vi "JSON to LVObject.vi"(7 "Class 1 in":refnum<class "Serializer-Palette.lvclass">, 8 "error in":errorcluster, 9 "Object Type":refnum<class>, 10 "Offset":i32, 11 "JSON":string) -> (0 "error out":errorcluster, 1 "Object":refnum<class>)   [LabVIEW 2021, in "TSC Material Theme.lvlib" / "Serializer-Palette.lvclass"]
doc: "Convert JSON to an Object of a LabVIEW Class."
uses:
  Serializer-Palette.lvclass
  Serializer-Palette.lvclass/Serializer-Palette.ctl
  TSC Material Theme/material json palette--cluster.ctl
  Material-Palette/Material-Palette.lvclass/Material-Palette.ctl
  TSC Material Theme/convert string to hex.vi
  Material-Palette/Material-Palette.lvclass
  <vilib>/JDP Science/JSONtext/JSONtext.lvlib
  TSC Material Theme/TSC Material Theme.lvlib
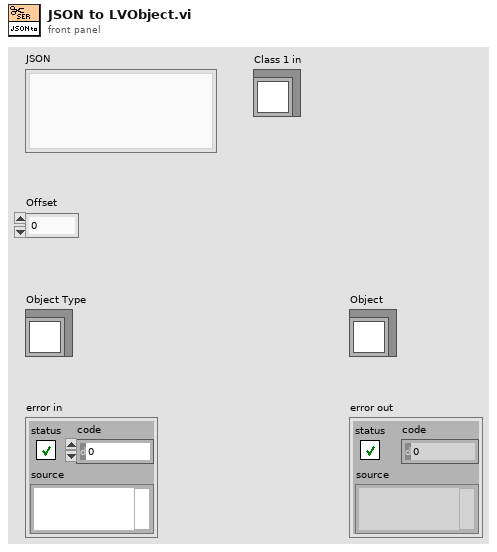
[diagram p1: front panel]
types:
  T1 = typedef "TSC Material Theme.lvlib/material json palette--cluster.ctl" = cluster{"0":string, "5":string, "10":string, "15":string, "20":string, "25":string, "30":string, "35":string, "40":string, "50":string, "60":string, "70":string, "80":string, "90":string, "95":string, "98":string, "99":string, "100":string}
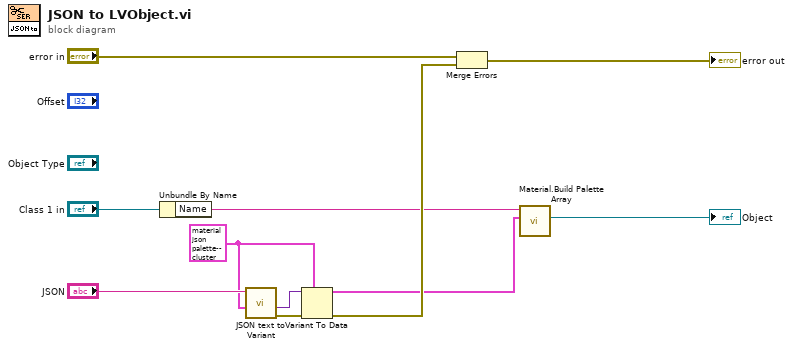
[diagram p0: block diagram]
diagram:
  w5 = T1 {"0"="", "5"="", "10"="", "15"="", "20"="", "25"="", "30"="", "35"="", "40"="", "50"="", "60"="", "70"="", "80"="", "90"="", "95"="", "98"="", "99"="", "100"=""} ("primary")
  n1 = Unbundle By Name("Class 1 in") -> ("Name"=w1:string)
  n2 = call <vilib>:"JSON text to Variant.vi"("Data Type"=w5, "JSON"="JSON") -> ("error out"=w11:errorcluster, "Variant out"=w6:variant)  [unwired: 8 in]
  n3 = Variant To Data(error in=w11, type=w5, Variant=w6) -> (data=w2:T1, error out=w9:errorcluster)
  n4 = Merge Errors("error in", w9) -> (→"error out":errorcluster)
  n5 = call "Material.Build Palette Array.vi"("palette"=w2, "Name"=w1) -> ("Palettes"=→"Object":refnum<class "Material-Palette.lvclass">)  [unwired: 9 in]
